vi "Update State.vi"(9 "New State":string, 10 "Process":string, 11 "Debug State Analyzer In":refnum<class "Debug State Analyzer.lvclass">) -> (3 "Debug State Analyzer Out":refnum<class "Debug State Analyzer.lvclass">)   [LabVIEW 2020, in "Debug State Analyzer.lvclass"]
uses:
  Debug State Analyzer.lvclass
  Debug State Analyzer.lvclass/Debug State Analyzer.ctl
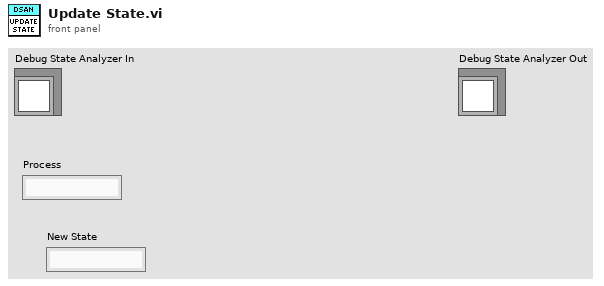
[diagram p1: front panel]
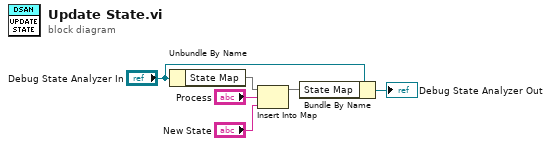
[diagram p0: block diagram]
diagram:
  n1 = Unbundle By Name("Debug State Analyzer In") -> ("State Map"=w3:map{string, string})
  n2 = Insert Into Map(map in=w3, key="Process", value="New State") -> (map out=w4:map{string, string})  [unwired: 2 out]
  n3 = Bundle By Name(cluster="Debug State Analyzer In", "State Map"=w4) -> (→"Debug State Analyzer Out":refnum<class "Debug State Analyzer.lvclass">)
